vi "write_config.vi"(0 "object in":refnum<class "interface.lvclass">, 5 "error in (no error)":errorcluster) -> (14 "object out":refnum<class "interface.lvclass">, 19 "error out":errorcluster)   [LabVIEW 2016, in "interface.lvclass"]
uses:
  interface.lvclass
  interface.lvclass/interface.ctl
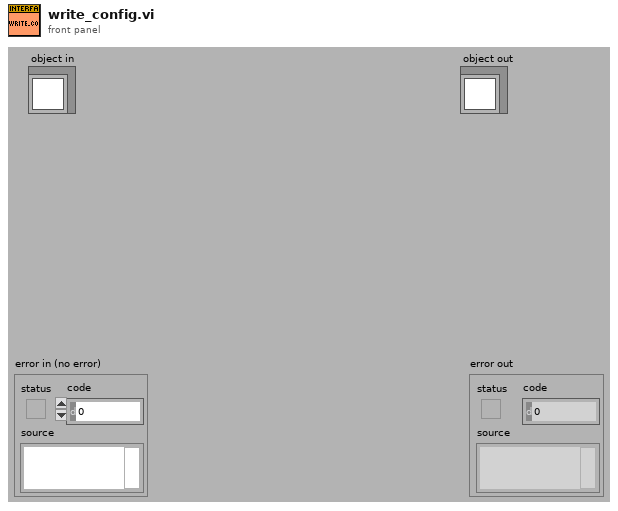
[diagram p1: front panel]
types:
  T1 = cluster{"updateconfiguration":refnum<vi>, "软件版本":refnum<vi>}
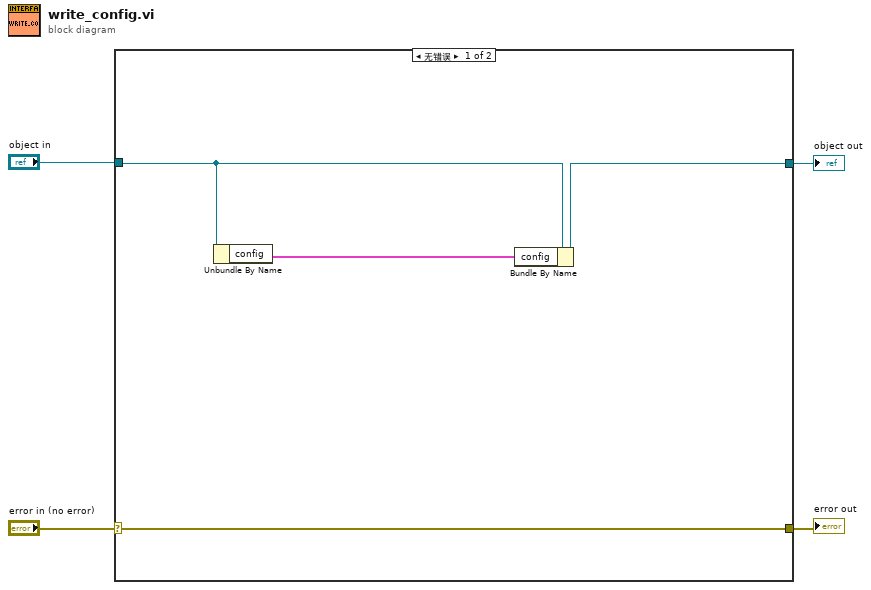
[diagram p0: block diagram]
diagram:
  n1 = case shown="无错误" "error in (no error)" {
    selector: "error in (no error)" -> [w7 w10]
    tunnel: [w7 w10] -> w3
    tunnel: [w5 w9] -> w1
    tunnel: "object in" -> [w6 w9]
    frame No Error {
      n2 = Unbundle By Name(w6) -> ("config"=w8:T1)
      n3 = Bundle By Name(cluster=w6, "config"=w8) -> (w5:refnum<class "interface.lvclass">)
    }
    frame Error {
    }
  }
  "error out" <- w3
  "object out" <- w1
